vi "command timer.vi"(7 "time (global)":dbl, 10 "time (next command)":dbl, 11 "command queue in":cluster{"Zeit [s]":i32, "Befehl":string}[](array[cluster])) -> (0 "Licor command":string, 2 "time (next command)":dbl, 3 "command queue out":cluster{"Zeit [s]":i32, "Befehl":string}[](array[cluster]))   [LabVIEW 2010]
panel:
  out "x-y":dbl
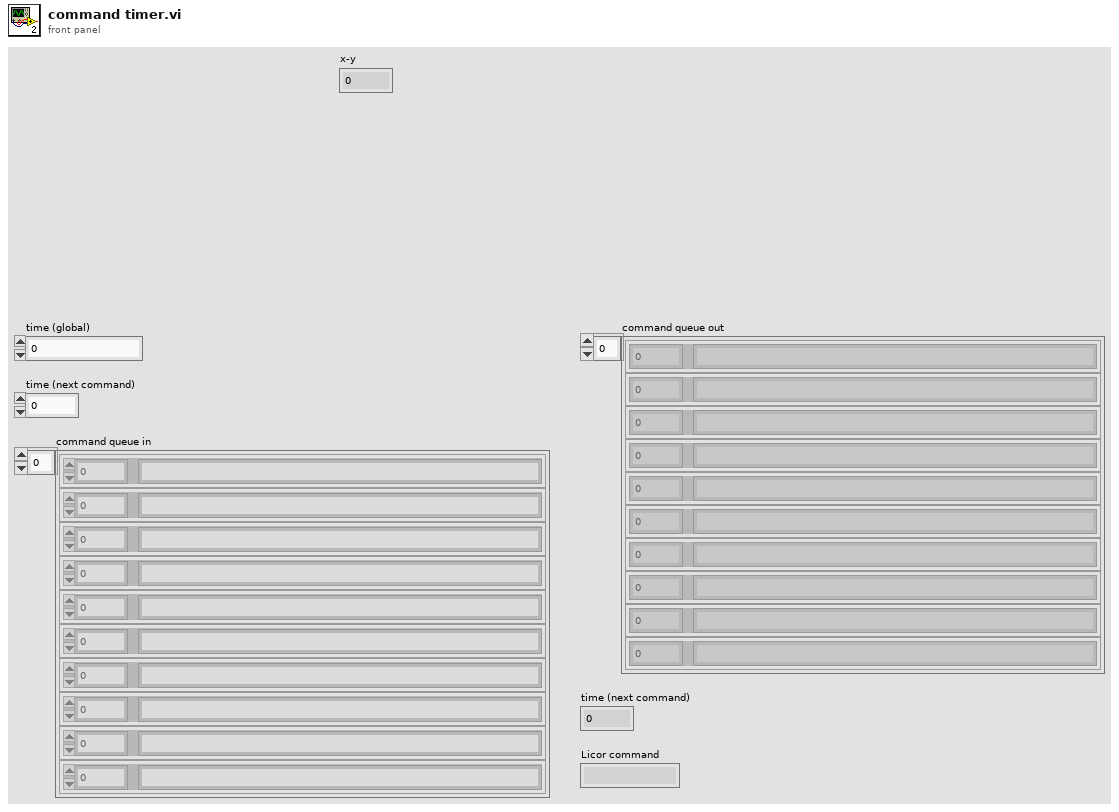
[diagram p1: front panel]
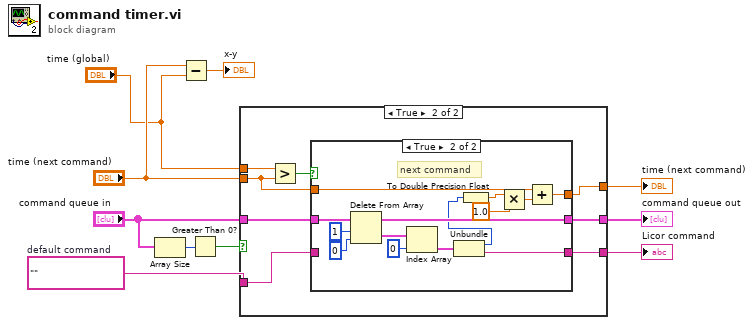
[diagram p0: block diagram]
diagram:
  w4 = ""  # default command
  n1 = Array Size(array="command queue in") -> (size(s)=w6:i32)
  n2 = Subtract(x="time (next command)", y="time (global)") -> (x-y=→"x-y":dbl)
  n3 = Greater Than 0?(x=w6) -> (x > 0?=w5:bool)
  n4 = case shown="True" w5 {
    tunnel: "time (global)" -> [w11 w21]
    tunnel: "time (next command)" -> [_ w19]
    tunnel: [w13 w18] -> w10
    tunnel: [w11 w17] -> w9
    tunnel: [w12 w16] -> w8
    tunnel: "command queue in" -> [w13 w15]
    tunnel: w4 -> [w12 w14]
    frame False {
      # "queue empty"
    }
    frame True {
      n5 = Greater?(x=w21, y=w19) -> (0:w20:bool)
      n6 = case shown="True" w20 {
        tunnel: w15 -> [w23 w37]
        tunnel: [w22 w32] -> w16
        tunnel: [w23 w31] -> w18
        tunnel: w19 -> [w24 w30]
        tunnel: [w24 w29] -> w17
        tunnel: w14 -> [w22 _]
        frame False {
          # "wait for next command"
        }
        frame True {
          # "next command"
          n7 = Delete From Array(array=w37, length=1 ("Länge"), index=0 ("Länge")) -> (deleted portion=w34:cluster{"Zeit [s]":i32, "Befehl":string}[], array with subset deleted=w31:cluster{"Zeit [s]":i32, "Befehl":string}[])
          n8 = Index Array(array=w34, index=0 ("Index")) -> (element=w33:cluster{"Zeit [s]":i32, "Befehl":string})
          n9 = Unbundle(w33) -> ("Zeit [s]"=w26:i32, "Befehl"=w32:string)
          n10 = To Double Precision Float(number=w26) -> (double precision float=w27:dbl)
          n11 = Multiply(x=w27, y=1.0) -> (x*y=w28:dbl)
          n12 = Add(x=w30, y=w28) -> (x+y=w29:dbl)
        }
      }
    }
  }
  "command queue out" <- w10
  "time (next command)" <- w9
  "Licor command" <- w8
